vi "Assert Log File Exists.vi"(8 "error in":errorcluster, 9 "message on error":string, 10 "file path":path=path "C:/logs/EDL2-archive/EDL Log2.tdms", 11 "Embedded Data Logger System Tests in":refnum<class "Embedded Data Logger Windows System Tests.lvclass">) -> (0 "error out":errorcluster, 3 "Embedded Data Logger System Tests out":refnum<class "Embedded Data Logger Windows System Tests.lvclass">)   [LabVIEW 2027, in "Embedded Data Logger Windows System Tests.lvclass"]
uses:
  Embedded Data Logger Windows System Tests.lvclass
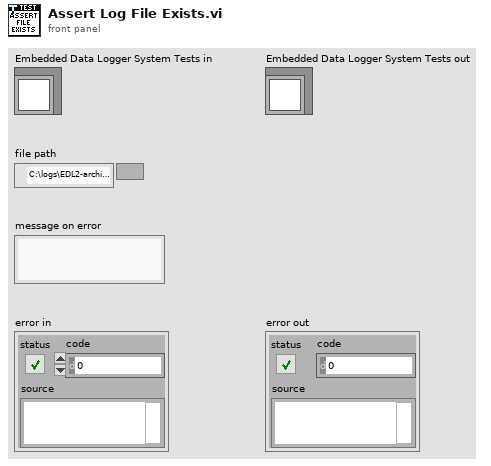
[diagram p1: front panel]
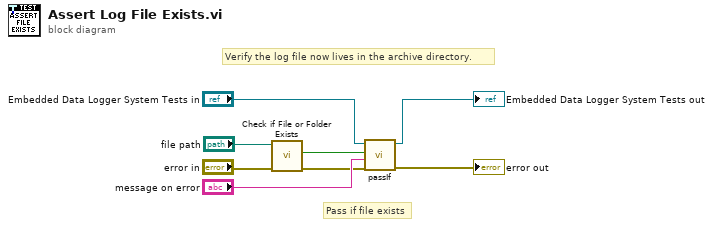
[diagram p0: block diagram]
diagram:
  # "Verify the log file now lives in the archive directory."
  # "Pass if file exists"
  n1 = call <vilib>:"Check if File or Folder Exists.vi"("error in (no error)"="error in", "path"="file path") -> ("error out"=w2:errorcluster, "file or folder exists?"=w1:bool)  [unwired: 7 in, 1 out]
  n2 = call-dynamic "passIf.vi"("error in (no error)"=w2, "message (\"\")"="message on error", "pass"=w1, "TestCase in"="Embedded Data Logger System Tests in") -> ("error out"=→"error out":errorcluster, "TestCase out"=→"Embedded Data Logger System Tests out":refnum<class "Embedded Data Logger Windows System Tests.lvclass">)  [unwired: 6 in]
